vi "random_no_array.vi"() -> ()   [LabVIEW 2015]
panel:
  out "Array":dbl[](array[numeric])
  out "Numeric":i32
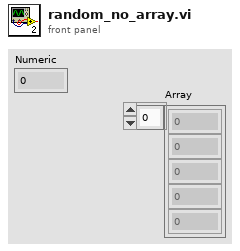
[diagram p1: front panel]
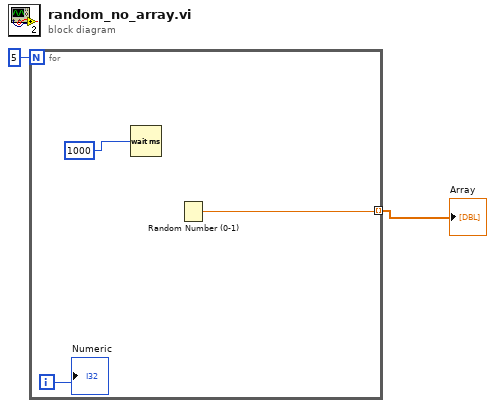
[diagram p0: block diagram]
diagram:
  n1 = for {
    N: 5 -> [_]
    tunnel: [w4] -> w1 mode=indexing
    i -> [w5]
    n2 = Wait (ms)(milliseconds to wait=u32 1000 ("millisecond timer value")) -> ()  [unwired: 1 out]
    n3 = Random Number (0-1)() -> (number: 0 to 1=w4:dbl)
    "Numeric" <- w5
  }
  "Array" <- w1
